vi "ProcessMatlabEvents.vi"(8 "Event Wait timeout":i32=5, 11 "ExpID":string="Exp967f258c607eed45caf40f4c3101458dC") -> ()   [LabVIEW 2017]
uses:
  Types/MatlabDataBundle.ctl
  Types/MatlabDataType.ctl
  Types/MatlabDataContainerType.ctl
  Types/MatlabBindingDirectionEnum.ctl
  Types/MethodInvokeInfo.ctl
panel:
  out "Number of events last read simultaniously":i32
  out "Reading events":bool
  out "Number of events read this round":i32
  out "InvokeDataChangedGlobalEvent":bool
  out "Checking changes on control":string="StreamingCounterState"
  out "Matlab Param Data":T1[](array[typedef])=[{"MatlabType"=enum."Boolean", "Value"=variant(bool FALSE), "Name"="", "Typename"="boolean", "Container Type"=enum."Numeric Value"}]
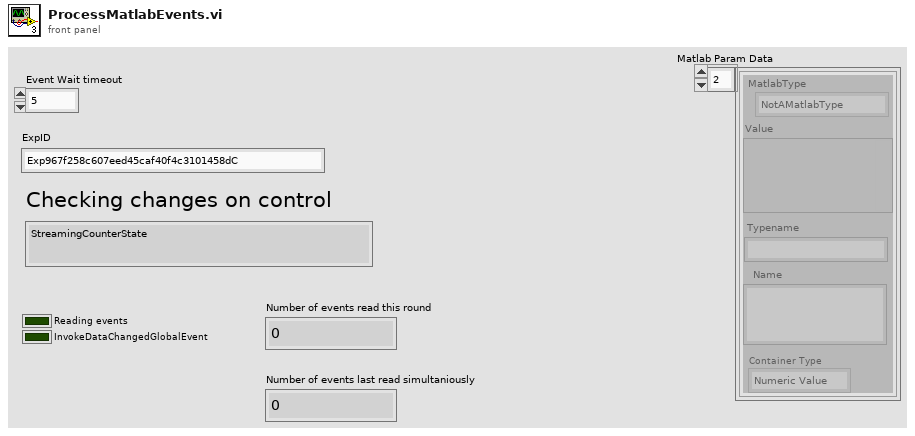
[diagram p1: front panel]
types:
  T1 = typedef "MatlabDataBundle.ctl" = cluster{"MatlabType":T2, "Value":variant, "Name":string, "Typename":string, "Container Type":T3}
  T2 = typedef "MatlabDataType.ctl" = enum16{"NotAMatlabType", "Real", "Complex", "String", "Boolean"}
  T3 = typedef "MatlabDataContainerType.ctl" = enum16{"Numeric Value", "Numeric Array", "Waveform"}
  T4 = typedef "MatlabBindingDirectionEnum.ctl" = enum16{"BiDirectional", "FromMatlab", "ToMatlab"}
  T5 = typedef "MethodInvokeInfo.ctl" = cluster{"Method Name":string, "Arguments":variant}
  T6 = typedef "ControlValueChangeEventBindingType.ctl" = cluster{"Control":refnum<vi>, "Event Register":refnum<event-registration>, "AllowVariantValues":bool, "Direction":T4, "Requires Update":bool, "Name":string}
  T7 = typedef "MatlabEventStruct.ctl" = cluster{"Name":string, "DataIndex":dbl, "Category":string, "Matlab Param Data":T1[]}
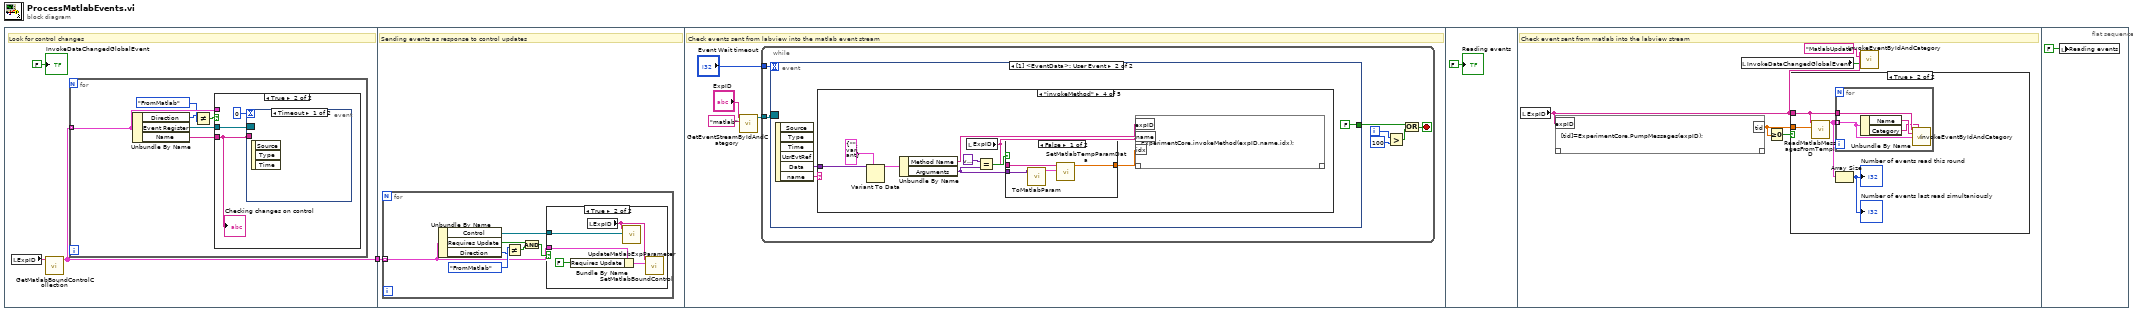
[diagram p0: block diagram]
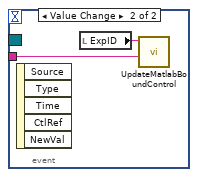
[diagram p3: hidden frame]
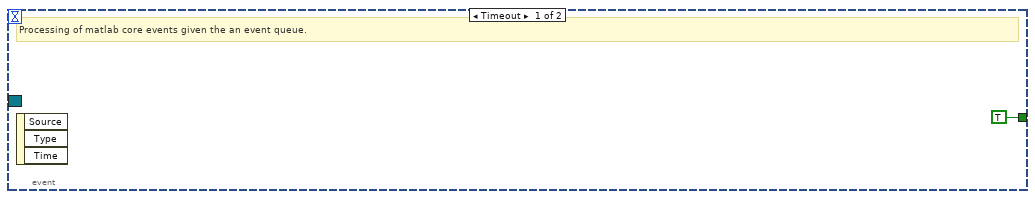
[diagram p5: hidden frame]
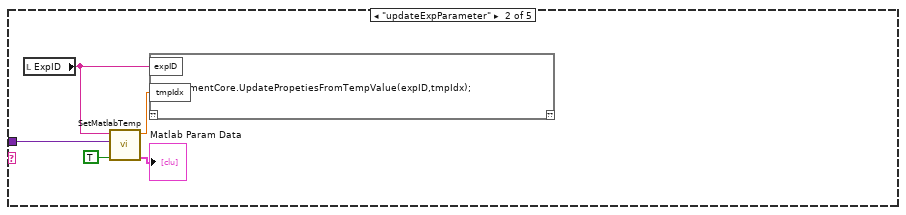
[diagram p7: hidden frame]
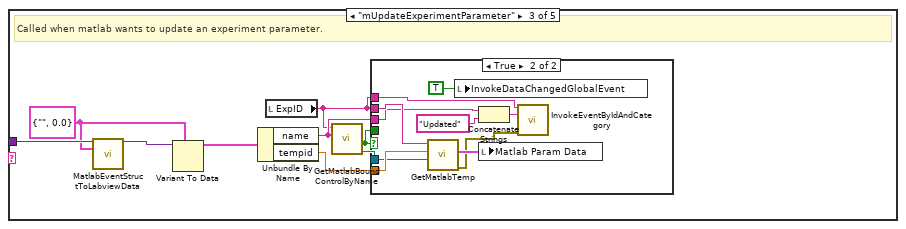
[diagram p8: hidden frame]
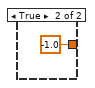
[diagram p10: hidden frame]
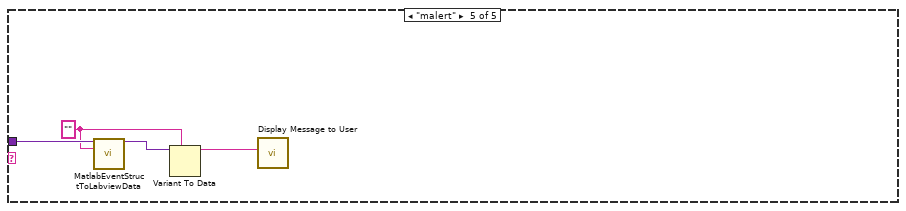
[diagram p11: hidden frame]
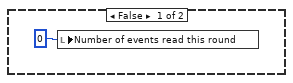
[diagram p12: hidden frame]
diagram:
  n1 = flat-sequence {
    tunnel: [w2] -> w1
    tunnel: w1 -> [w16]
    frame #0 {
      # "Look for control changes"
      n2 = local read "ExpID"() -> (w4:string)
      n3 = call "GetMatlabBoundControlCollection.vi"("ExpID"=w4) -> ("Bound Controls"=w2:T6[])  [unwired: 10 in]
      n4 = for {
        tunnel: w2 -> [w10] mode=indexing
        n5 = Unbundle By Name(w10) -> ("Direction"=w7:T4, "Event Register"=w6:refnum<event-registration>, "Name"=w5:string)
        n6 = Not Equal?(x=w7, y=MatlabBindingDirectionEnum."FromMatlab" ("Direction")) -> (x != y?=w8:bool)
        n7 = case shown="True" w8 {
          tunnel: w10 -> [_ _]
          tunnel: w6 -> [_ w12]
          tunnel: w5 -> [_ w11]
          frame False {
          }
          frame True {
            n8 = event shown="[0] Timeout" {
              selector: w12 -> [_ _]
              dyn-events: _ -> [_ _]
              timeout: 0 -> [_ _]
              tunnel: w11 -> [_ w14]
              event Timeout {
                n9 = event-data() -> ()  [unwired: 1 in, 3 out]
              }
              event Value Change {
                n10 = event-data() -> ()  [unwired: 1 in, 5 out]
                n11 = local read "ExpID"() -> (w15:string)
                n12 = call "UpdateMatlabBoundControl.vi"("name"=w14, "ExpID"=w15) -> ()  [unwired: 10 in]
              }
            }
            "Checking changes on control" <- w11
          }
        }
      }
      "InvokeDataChangedGlobalEvent" <- FALSE ("InvokeDataChangedGlobalEvent")
    }
    frame #1 {
      # "Sending events as response to control updates"
      n13 = for {
        tunnel: w16 -> [w17] mode=indexing
        n14 = Unbundle By Name(w17) -> ("Control"=w18:refnum<vi>, "Requires Update"=w19:bool, "Direction"=w21:T4)
        n15 = Not Equal?(x=MatlabBindingDirectionEnum."FromMatlab" ("Direction"), y=w21) -> (x != y?=w20:bool)
        n16 = And(x=w19, y=w20) -> (x .and. y?=w23:bool)
        n17 = case shown="True" w23 {
          tunnel: w18 -> [_ w28]
          tunnel: w17 -> [_ w27]
          frame False {
          }
          frame True {
            n18 = Bundle By Name(cluster=w27, "Requires Update"=FALSE) -> (w24:T6)
            n19 = local read "ExpID"() -> (w25:string)
            n20 = call "UpdateMatlabExpParameter.vi"("Parameter(s)"=w28, "ExpID"=w25) -> ()  [unwired: 9 in, 1 out]
            n21 = call "SetMatlabBoundControl.vi"("Control Binding"=w24, "ExperimentID"=w25) -> ()  [unwired: 10 in]
          }
        }
      }
    }
    frame #2 {
      # "Check events sent from labview into the matlab event stream"
      n22 = call "GetEventStreamByIdAndCategory.vi"("Category"="matlab", "ID"="ExpID") -> ("Event Registration Refnum out"=w30:refnum<event-registration>)  [unwired: 7 in, 2 out]
      n23 = while {
        tunnel: w30 -> [w39]
        tunnel: "Event Wait timeout" -> [w38]
        i -> [w37]
        stop <- w34 stop-if-true
        n24 = event shown="[1] <EventData>: User Event" {
          selector: w39 -> [_ _]
          dyn-events: _ -> [_ _]
          timeout: w38 -> [_ _]
          tunnel: [TRUE FALSE] -> w33
          event Timeout {
            # "Processing of matlab core events given the an event queue."
            n25 = event-data() -> ()  [unwired: 1 in, 3 out]
          }
          event User Event {
            n26 = event-data() -> ("Data"=w42:variant, "name"=w43:string)  [unwired: 1 in, 4 out]
            n27 = case shown="\"invokeMethod\"" w43 {
              tunnel: w42 -> [_ w46 w56 w75 w85]
              frame "False", Default {
              }
              frame "updateExpParameter" {
                n28 = local read "ExpID"() -> (w48:string)
                n29 = call "SetMatlabTemp.vi"("Add Container Name? (f)"=TRUE, "Variant"=w46, "ExpID"=w48) -> ("Matlab Param Data"=→"Matlab Param Data":T1[], "Temp Index"=w47:dbl)  [unwired: 7 in]
                n30 = script code="ExperimentCore.UpdatePropetiesFromTempValue(expID,tmpIdx);"("expID"=w48, "tmpIdx"=w47) -> ()  [unwired: 1 in, 1 out]
              }
              frame "mUpdateExperimentParameter" {
                w55 = cluster{"name":string, "tempid":dbl} {"name"="", "tempid"=0.0}
                # "Called when matlab wants to update an experiment parameter."
                n31 = call "MatlabEventStructToLabviewData.vi"("Event Variant"=w56, "Value to update (or object type)"=w55) -> ("Value"=w57:variant)  [unwired: 11 in, 2 out]
                n32 = Variant To Data(type=w55, Variant=w57) -> (data=w54:cluster{"name":string, "tempid":dbl})  [unwired: 1 in, 1 out]
                n33 = Unbundle By Name(w54) -> ("name"=w50:string, "tempid"=w53:dbl)
                n34 = local read "ExpID"() -> (w49:string)
                n35 = call "GetMatlabBoundControlByName.vi"("name"=w50, "ExperimentID"=w49) -> ("Control"=w52:refnum<vi>, "found"=w51:bool)  [unwired: 7 in, 1 out]
                n36 = case shown="True" w51 {
                  tunnel: w53 -> [_ w67]
                  tunnel: w49 -> [_ w65]
                  tunnel: w51 -> [_ _]
                  tunnel: w52 -> [_ w63]
                  tunnel: w50 -> [_ w61]
                  tunnel: w49 -> [_ w59]
                  frame False {
                  }
                  frame True {
                    n37 = call "GetMatlabTemp.vi"("Value To Update (or type)"=w63, "index in"=w67, "ExpID"=w65) -> ("error out"=w58:errorcluster, "Matlab param data"=w66:T1[])  [unwired: 6 in, 1 out]
                    n38 = local write "InvokeDataChangedGlobalEvent"(TRUE ("InvokeDataChangedGlobalEvent")) -> ()
                    n39 = Concatenate Strings(w61, "Updated" ("eventName")) -> (w62:string)
                    n40 = local write "Matlab Param Data"(w66) -> ()
                    n41 = call "InvokeEventByIdAndCategory.vi"("ID"=w59, "eventName"=w62, "error in (no error)"=w58) -> ()  [unwired: 12 in, 1 out]
                  }
                }
              }
              frame "invokeMethod" {
                n42 = Variant To Data(type=T5 {"Method Name"="", "Arguments"=variant} ("Method Invoke Info"), Variant=w75) -> (data=w74:T5)  [unwired: 1 in, 1 out]
                n43 = Unbundle By Name(w74) -> ("Method Name"=w69:string, "Arguments"=w70:variant)
                n44 = local read "ExpID"() -> (w68:string)
                n45 = Equal?(x=variant, y=w70) -> (x = y?=w71:bool)
                n46 = case shown="False" w71 {
                  tunnel: [w78 -1.0] -> w72
                  tunnel: w70 -> [w79 _]
                  tunnel: w68 -> [w77 _]
                  frame False {
                    n47 = call "ToMatlabParam.vi"("Value"=w79) -> ("Matlab Param Data"=w80:T1[])  [unwired: 10 in]
                    n48 = call "SetMatlabTempParamData.vi"("Matlab param data"=w80, "ExperimentID"=w77) -> ("index out"=w78:dbl)  [unwired: 9 in]
                  }
                  frame True {
                  }
                }
                n49 = script code="ExperimentCore.invokeMethod(expID,name,idx);"("expID"=w68, "name"=w69, "idx"=w72) -> ()  [unwired: 1 in, 1 out]
              }
              frame "malert" {
                w82 = ""
                n50 = call "MatlabEventStructToLabviewData.vi"("Event Variant"=w85, "Value to update (or object type)"=w82) -> ("Value"=w84:variant)  [unwired: 11 in, 2 out]
                n51 = Variant To Data(type=w82, Variant=w84) -> (data=w83:string)  [unwired: 1 in, 1 out]
                n52 = call "Display Message to User"("Message"=w83) -> ()  [unwired: 9 in, 2 out]
              }
            }
          }
        }
        n53 = Greater?(x=w37, y=100) -> (0:w35:bool)
        n54 = Or(x=w33, y=w35) -> (x .or. y?=w34:bool)
      }
    }
    frame #3 {
      "Reading events" <- FALSE ("Reading events")
    }
    frame #4 {
      # "Check event sent from matlab into the labview stream"
      n55 = local read "ExpID"() -> (w89:string)
      n56 = script code="[tid]=ExperimentCore.PumpMessages(expID);"("expID"=w89) -> ("tid"=w91:dbl)  [unwired: 1 in, 1 out]
      n57 = local read "InvokeDataChangedGlobalEvent"() -> (w87:bool)
      n58 = Greater Or Equal To 0?(x=w91) -> (x >= 0?=w90:bool)
      n59 = case shown="True" w90 {
        tunnel: w91 -> [_ w96]
        tunnel: w89 -> [_ w95]
        frame False {
          n60 = local write "Number of events read this round"(0 ("Number of events read")) -> ()
        }
        frame True {
          n61 = call "ReadMatlabMessagesFromTempID.vi"("Numeric"=w96, "ExperimentID"=w95) -> ("Read messages"=w94:T7[])  [unwired: 9 in]
          n62 = for {
            tunnel: w94 -> [w98] mode=indexing
            tunnel: w95 -> [w100]
            n63 = Unbundle By Name(w98) -> ("Name"=w99:string, "Category"=w97:string)
            n64 = call "InvokeEventByIdAndCategory.vi"("ID"=w100, "Category"=w97, "eventName"=w99, "Data"=w98) -> ()  [unwired: 11 in, 1 out]
          }
          n65 = Array Size(array=w94) -> (size(s)=→"Number of events read this round" →"Number of events last read simultaniously":i32)
        }
      }
      n66 = call "InvokeEventByIdAndCategory.vi"("ID"=w89, "eventName"="MatlabUpdate", "Invoke? (t)"=w87) -> ()  [unwired: 12 in, 1 out]
    }
    frame #5 {
      n67 = local write "Reading events"(FALSE ("Reading events")) -> ()
    }
  }
